vi "HFRR ADV v06.vi"() -> ()   [LabVIEW 2025] (continued)
                  n763 = property class="Instr"(reference=w1044, error in=w1045) -> (reference out=w1049:refnum<visa-resource-name>, error out=w1048:errorcluster, "Serial Settings:Number of Bytes at Serial Port"=w1040:u32)
                  n764 = VISA Read(VISA resource name=w1049, byte count=w1040, error in (no error)=w1048) -> (VISA resource name out=w1046:refnum<visa-resource-name>, read buffer=w1038:string, error out=w1047:errorcluster)  [unwired: 1 out]
                  n765 = Greater?(x=w1040, y=u32 30) -> (0:w1042:bool)
                  n766 = Concatenate Strings(w1039, w1038) -> (w1037:string)
                }
                "UnoRead" <- w989
                n767 = while {
                  shift-right: [w1023] -> w1000
                  shift-left: w989 -> [w1029]
                  tunnel: [w1022] -> w996 mode=indexing
                  tunnel: [w1024] -> _
                  i -> [w1024]
                  stop <- w1026 stop-if-true
                  n768 = Match Pattern(string=w1029, regular expression="*") -> (after substring=w1027:string)  [unwired: 1 in, 3 out]
                  n769 = Match Pattern(string=w1027, regular expression="&") -> (before substring=w1022:string, after substring=w1023:string, offset past match=w1025:i32)  [unwired: 1 in, 1 out]
                  n770 = Less Than 0?(x=w1025) -> (x < 0?=w1026:bool)
                }
                n771 = local write "Residual Uno"(w1000) -> ()
                n772 = Array Size(array=w996) -> (size(s)=w997:i32)
                n773 = Decrement(x=w997) -> (x-1=w999:i32)
                n774 = Delete From Array(array=w996, length=1, index=w999) -> (array with subset deleted=w994:string[])  [unwired: 1 out]
                n775 = Array Size(array=w994) -> (size(s)=w993:i32)
                n776 = Decrement(x=w993) -> (x-1=w992:i32)
                n777 = while {
                  tunnel: [w1021] -> w1005 mode=indexing
                  tunnel: [w1020] -> w1004 mode=indexing
                  tunnel: w994 -> [w1014] mode=indexing
                  tunnel: w992 -> [w1013]
                  tunnel: [w1011] -> _
                  i -> [w1011]
                  stop <- w1012 stop-if-true
                  w1015 = 0 ("length (rest)")
                  w1017 = ";" ("regular expression")
                  n778 = Less Or Equal?(x=w1013, y=w1011) -> (x <= y?=w1012:bool)
                  n779 = Match Pattern(string=w1014, regular expression=w1017) -> (before substring=w1019:string, after substring=w1018:string)  [unwired: 1 in, 2 out]
                  n780 = Decimal String To Number(string=w1019, default (0L)=w1015) -> (number=w1021:i32)  [unwired: 1 in, 1 out]
                  n781 = Match Pattern(string=w1018, regular expression=w1017) -> (before substring=w1016:string)  [unwired: 1 in, 3 out]
                  n782 = Decimal String To Number(string=w1016, default (0L)=w1015) -> (number=w1020:i32)  [unwired: 1 in, 1 out]
                }
                n783 = case shown="0, Default" "ADC Res" {
                  tunnel: [w1032 w1034] -> w988
                  frame 0, Default {
                    n784 = Divide(x=65535 ("length (rest)"), y=2 ("length (rest)")) -> (x/y=w1032:dbl)
                  }
                  frame 1 {
                    n785 = Divide(x=16777216 ("length (rest)"), y=2 ("length (rest)")) -> (x/y=w1034:dbl)
                  }
                }
                n786 = Bundle(w1005, w1004) -> (w995:cluster{i32[], i32[]})  [unwired: 1 in]
                n787 = Divide(x=w995, y=w988) -> (x/y=w1006:cluster{dbl[], dbl[]})
                n788 = Multiply(x=w1006, y=sgl 5.03 ("Numeric")) -> (x*y=w1003:cluster{dbl[], dbl[]})
                n789 = Unbundle(w1003) -> (→"Ch1":dbl[], →"Ch0":dbl[])
              }
            }
            n790 = Not(x=w977) -> (.not. x?=→"Port 1a":bool)
          }
          frame #1 {
            n791 = local read "zOff 2"() -> (w1084:dbl)
            n792 = local read "Ch1"() -> (w1074:dbl[])
            n793 = case shown="True" "Zero 2" {
              tunnel: w1074 -> [_ w1104]
              frame False {
              }
              frame True {
                n794 = call-poly <vilib>:"Mean.vi"("X"=w1104) -> ("mean"=→"zOff 2":dbl)  [unwired: 1 out]
                n795 = local write "Zero 2"(FALSE ("Zero")) -> ()
              }
            }
            n796 = Subtract(x=w1074, y=w1084) -> (x-y=w1080:dbl[])
            n797 = call-poly <vilib>:"Mean.vi"("X"=w1074) -> ("mean"=w1075:dbl)  [unwired: 1 out]
            "Slide 3" <- w1075
            n798 = Multiply(x=w1080, y=1.0 ("PG Oth")) -> (x*y=w1066:dbl[])
            n799 = local read "FF buffer"() -> (w1071:dbl[])
            n800 = Divide(x=w1066, y=1) -> (x/y=w1065:dbl[])
            "Fric Val" <- w1065
            n801 = call <vilib>:"Mean PtByPt.vi"("x"=w1075, "sample length"=10, "initialize"="Reset 2") -> ("mean"=→"Mean Pos Fil 2":dbl)  [unwired: 1 in, 1 out]
            n802 = Array Size(array=w1071) -> (size(s)=w1073:i32)
            n803 = call-poly <vilib>:"Mean.vi"("X"=w1065) -> ("mean"=w1079:dbl)  [unwired: 1 out]
            n804 = Insert Into Array(array=w1071, index=w1073, new element=w1065) -> (w1068:dbl[])
            n805 = Array Size(array=w1068) -> (size(s)=w1067:i32)
            n806 = case shown="True" "DC corr 2" {
              tunnel: w1065 -> [w1107 w1110]
              tunnel: [w1107 w1109] -> w1072
              tunnel: w1079 -> [_ w1108]
              frame False {
              }
              frame True {
                n807 = Subtract(x=w1110, y=w1108) -> (x-y=w1109:dbl[])
              }
            }
            n808 = Tick Count (ms)() -> (millisecond timer value=w1091:u32)
            n809 = Greater?(x=w1067, y=1000) -> (0:w1069:bool)
            n810 = Subtract(x=w1091, y=w1092) -> (x-y=w1090:u32)
            n811 = case shown="True" w1069 {
              tunnel: [w1097 w1100] -> w1056
              tunnel: w1068 -> [w1097 w1103]
              tunnel: w1067 -> [_ w1102]
              frame False {
              }
              frame True {
                n812 = Subtract(x=w1102, y=1000) -> (x-y=w1098:i32)
                n813 = Delete From Array(array=w1103, length=w1098, index=0) -> (array with subset deleted=w1100:dbl[])  [unwired: 1 out]
              }
            }
            n814 = Divide(x=w1090, y=u32 1000 ("x")) -> (x/y=w1088:dbl)
            n815 = Array Size(array=w1072) -> (size(s)=w1087:i32)
            n816 = Divide(x=w1087, y=w1088) -> (x/y=w1083:dbl)
            "Sps 2" <- w1083
            n817 = Reciprocal(x=w1083) -> (1/x=w1081:dbl)
            "dt" <- w1081
            n818 = local read "FRIC. FORCE :"() -> (w1053:dbl)
            n819 = local write "FF buffer"(w1056) -> ()
            n820 = Negate(x=w1056) -> (-x=w1055:dbl[])
            n821 = call "Elapsed Time5"("Time Target (s)"="check time s", "Reset"="Reset 3") -> ("Time has Elapsed"=w1058:bool)  [unwired: 10 in, 7 out]
            n822 = Array Max & Min(array=w1055) -> (max value=w1063:dbl)  [unwired: 3 out]
            n823 = Bundle By Name("Y"=w1072, "dt"=w1081, "t0"=timestamp(0 s since 1904-01-01)) -> (w1051:waveform(dbl))  [unwired: 1 in]
            n824 = Multiply(x=w1053, y=21.1986) -> (x*y=w1052:dbl)
            n825 = Greater Or Equal?(x=w1063, y="Threshold value") -> (x >= y?=w1059:bool)
            n826 = Multiply(x=w1052, y=w1051) -> (x*y=→"FF_Wfm":waveform(dbl))
            n827 = And(x=w1059, y=w1058) -> (x .and. y?=w1057:bool)
            n828 = case shown="True" w1057 {
              frame False {
                n829 = local write "Reset 3"(FALSE ("Reset 3")) -> ()
              }
              frame True {
                n830 = local write "Reset 3"(TRUE ("Reset 3")) -> ()
                n831 = local write "save dpt"(TRUE ("save dpt")) -> ()
              }
            }
          }
          frame #2 {
            n832 = local read "FF buffer"() -> (w1117:dbl[])
            n833 = Array Max & Min(array=w1117) -> (max value=w1112:dbl, min value=w1113:dbl)  [unwired: 2 out]
            n834 = Subtract(x=w1112, y=w1113) -> (x-y=w1114:dbl)
            n835 = Multiply(x=1.0 ("y 2"), y="Threshold") -> ()  [unwired: 1 out]
            n836 = Greater?(x=w1114, y="Threshold") -> (0:w1111:bool)
            n837 = case shown="True" w1111 {
              tunnel: w1117 -> [_ w1124]
              tunnel: [_ w1122] -> _
              frame False {
              }
              frame True {
                w1123 = 1.0 ("y")
                n838 = Delete From Array(array=w1124, length=100, index=0) -> (deleted portion=w1129:dbl[])  [unwired: 1 out]
                n839 = call-poly <vilib>:"Mean.vi"("X"=w1129) -> ("mean"=w1128:dbl)  [unwired: 1 out]
                n840 = Subtract(x=w1124, y=w1128) -> (x-y=w1127:dbl[])
                n841 = Multiply(x=w1123, y=w1123) -> (x*y=w1125:dbl)
                n842 = Multiply(x=w1127, y=w1125) -> (x*y=w1126:dbl[])
                "FF cal val" <- w1126
                n843 = Array Size(array=w1126) -> (size(s)=w1120:i32)
                n844 = Array Max & Min(array=w1126) -> (max value=w1119:dbl, min value=w1118:dbl)  [unwired: 2 out]
                n845 = property on="FF Calibration g" class="WFGraph (strict)"("X Scale.Range:Minimum"=0.0 ("y"), "X Scale.Range:Maximum"=w1120, "Y Scale.Range:Minimum"=w1119, "Y Scale.Range:Maximum"=w1118) -> ()  [unwired: 2 in, 2 out]
                n846 = local read "FRIC. FORCE :"() -> (w1122:dbl)
              }
            }
          }
          frame #3 {
            # "5"
            n847 = local read "DISPLACEMENT :"() -> (w1217:dbl)
            n848 = Multiply(x=w1217, y=1.0) -> (x*y=w1134:dbl)
            n849 = local read "zOff 3"() -> (w1220:dbl)
            n850 = local read "Ch0"() -> (w1147:dbl[])
            n851 = case shown="True" "Zero 3" {
              tunnel: w1147 -> [_ w1235]
              frame False {
              }
              frame True {
                n852 = call-poly <vilib>:"Mean.vi"("X"=w1235) -> ("mean"=→"zOff 3":dbl)  [unwired: 1 out]
                n853 = local write "Zero 3"(FALSE ("Zero")) -> ()
              }
            }
            n854 = Add(x=w1147, y="Offset") -> (x+y=w1146:dbl[])
            n855 = Multiply(x=w1134, y="DISPLACEMENT : 2") -> (x*y=w1201:dbl)
            n856 = Subtract(x=w1147, y=w1220) -> (x-y=w1204:dbl[])
            n857 = Multiply(x=w1204, y=w1201) -> (x*y=w1203:dbl[])
            n858 = Multiply(x=w1204, y=w1134) -> (x*y=w1216:dbl[])
            "ABS DP" <- w1216
            n859 = local read "Standard Slip Gauge (mm)"() -> (w1202:dbl)
            n860 = call-poly <vilib>:"Mean.vi"("X"=w1203) -> ("mean"=w1133:dbl)  [unwired: 1 out]
            "Disp (mm)" <- w1133
            "software msrnt" <- w1133
            n861 = Multiply(x=w1146, y="Gain") -> (x*y=w1141:dbl[])
            "Voltage LVDT Acq" <- w1141
            "gLVDTraw" <- w1141
            n862 = call-poly <vilib>:"Mean.vi"("X"=w1216) -> ("mean"=w1206:dbl)  [unwired: 1 out]
            n863 = case shown="True" "DC correction" {
              tunnel: w1216 -> [w1238 w1241]
              tunnel: [w1238 w1240] -> w1153
              tunnel: w1206 -> [_ w1239]
              frame False {
              }
              frame True {
                n864 = Subtract(x=w1241, y=w1239) -> (x-y=w1240:dbl[])
              }
            }
            n865 = Divide(x=w1133, y=w1202) -> (x/y=w1200:dbl)
            n866 = call-poly <vilib>:"Mean.vi"("X"=w1141) -> ("mean"=w1140:dbl)  [unwired: 1 out]
            n867 = Array Max & Min(array=w1141) -> (max value=w1145:dbl, min value=w1144:dbl)  [unwired: 2 out]
            n868 = Multiply(x=w1200, y=w1201) -> (x*y=→"DISPLACEMENT : 3":dbl)
            n869 = Subtract(x=w1145, y=w1144) -> (x-y=→"Pk-Pk":dbl)
            n870 = local read "dt"() -> (w1219:dbl)
            n871 = Threshold 1D Array(2:0.0 ("threshold y"), 3:w1153) -> (0:w1170:dbl)  [unwired: 1 in]
            n872 = Bundle By Name("Y"=w1153, "dt"=w1219, "t0"=timestamp(0 s since 1904-01-01)) -> (w1208:waveform(dbl))  [unwired: 1 in]
            n873 = local read "FF_Wfm"() -> (w1207:waveform(dbl))
            n874 = Equal To 0?(x=w1170) -> (x = 0?=w1171:bool)
            n875 = case shown="True" w1171 {
              tunnel: w1153 -> [_ w1229]
              tunnel: [w1225 w1226] -> w1166
              tunnel: w1170 -> [w1225 _]
              frame False {
              }
              frame True {
                n876 = Threshold 1D Array(1:20 ("start index (0)"), 2:0.0 ("threshold y"), 3:w1229) -> (0:w1226:dbl)
              }
            }
            n877 = call-poly <vilib>:"Extract Single Tone Information.vi"("time signal in"=w1208) -> ("detected amplitude"=w1142:dbl, "detected frequency"=→"Freq":dbl)  [unwired: 5 in, 4 out]
            n878 = Build Array(w1208, w1207) -> (w1189:waveform(dbl)[])
            "Waveform Graph 2" <- w1189
            n879 = Subtract(x=w1140, y="LvdtOff") -> (x-y=w1139:dbl)
            n880 = Subtract(x=w1139, y=w1142) -> (x-y=w1151:dbl)
            n881 = Add(x=w1142, y=w1139) -> (x+y=w1150:dbl)
            n882 = Index Array(array=w1189) -> (element #1=w1190:waveform(dbl), element #2=w1192:waveform(dbl))  [unwired: 2 in]
            n883 = Multiply(x=w1142, y=2.0) -> (x*y=w1209:dbl)
            "Stroke" <- w1209
            "Mean(RAW) Stroke" <- w1209
            n884 = Bundle(w1139, w1151, w1150) -> (→"Slide 8":cluster{dbl, dbl, dbl})  [unwired: 1 in]
            n885 = Unbundle By Name(w1190) -> ("Y"=w1163:dbl[])
            n886 = Split 1D Array(array=w1153, index=w1166) -> (second subarray=w1167:dbl[])  [unwired: 1 out]
            n887 = In Range and Coerce(upper limit=1.5, x=w1209, lower limit=0.5) -> (In Range?=w1213:bool)  [unwired: 1 out]
            n888 = Split 1D Array(array=w1163, index="Window") -> (second subarray=w1181:dbl[])  [unwired: 1 out]
            n889 = Unbundle By Name(w1192) -> ("Y"=w1164:dbl[])
            n890 = Threshold 1D Array(1:180 ("start index (0)"), 2:0.0 ("threshold y"), 3:w1167) -> (0:w1165:dbl)
            n891 = local read "Test \nStatus"() -> (w1210:bool)
            n892 = Split 1D Array(array=w1164, index=w1166) -> (second subarray=w1161:dbl[])  [unwired: 1 out]
            n893 = Not(x=w1213) -> (.not. x?=w1212:bool)
            n894 = call-poly <vilib>:"RMS.vi"("X"=w1181) -> ("rms value"=w1137:dbl)  [unwired: 1 out]
            "Current (A)" <- w1137
            n895 = Array Max & Min(array=w1181) -> (max value=w1195:dbl, min value=w1196:dbl)  [unwired: 2 out]
            n896 = Array Max & Min(array=w1164) -> (max value=w1193:dbl, min value=w1194:dbl)  [unwired: 2 out]
            n897 = Subtract(x=w1195, y=w1196) -> (x-y=w1197:dbl)
            n898 = Subtract(x=w1193, y=w1194) -> (x-y=w1198:dbl)
            n899 = And(x=w1212, y=w1210) -> (x .and. y?=w1211:bool)
            n900 = Split 1D Array(array=w1167, index=w1165) -> (first subarray=w1160:dbl[])  [unwired: 1 out]
            n901 = Split 1D Array(array=w1161, index=w1165) -> (first subarray=w1158:dbl[])  [unwired: 1 out]
            n902 = case shown="True" w1211 {
              tunnel: [i32[] [] w1231] -> _
              frame False {
              }
              frame True {
                n903 = local read "UnoRead"() -> (w1233:string)
                n904 = local read "Array"() -> (w1234:string[])
                n905 = Build Array (concatenate)(w1234, w1233) -> (w1232:string[])
                "Array" <- w1232
                n906 = String Length(string=w1232) -> (length=w1231:i32[])
              }
            }
            n907 = local read "G_val"() -> (w1183:dbl)
            n908 = Divide(x=w1198, y=w1197) -> (x/y=w1186:dbl)
            n909 = call-poly <vilib>:"RMS.vi"("X"=w1158) -> ("rms value"=w1182:dbl)  [unwired: 1 out]
            n910 = call-poly <vilib>:"Hanning Window.vi"("X"=w1160) -> ("Windowed X"=w1159:dbl[])  [unwired: 1 out]
            n911 = call-poly <vilib>:"Hanning Window.vi"("X"=w1158) -> ("Windowed X"=w1157:dbl[])  [unwired: 1 out]
            n912 = local read "Constant (G)"() -> (w1175:dbl)
            n913 = Divide(x=w1182, y=w1137) -> (x/y=w1176:dbl)
            n914 = Build Array(w1159, w1157) -> (→"Waveform Graph 4":dbl[][])
            n915 = Multiply(x=w1186, y=0.2) -> (x*y=w1188:dbl)
            n916 = Multiply(x=0.8 ("y"), y=w1183) -> (x*y=w1187:dbl)
            n917 = Add(x=w1188, y=w1187) -> (x+y=w1155:dbl)
            n918 = Multiply(x=w1176, y=0.2) -> (x*y=w1177:dbl)
            n919 = Multiply(x=0.8 ("y"), y=w1175) -> (x*y=w1178:dbl)
            n920 = Add(x=w1177, y=w1178) -> (x+y=w1174:dbl)
            "Constant (G)" <- w1174
            n921 = Not A Number/Path/Refnum?(number/path/refnum=w1155) -> (NaN/Path/Refnum?=w1154:bool)
            n922 = Select(t=0.0, s=w1154, f=w1155) -> (s? t:f=w1135:dbl)
            "G_val" <- w1135
            n923 = Multiply(x=w1137, y=w1135) -> (x*y=→"Friction Force (N)":dbl)
            n924 = Bundle(w1174, "t"=w1135) -> (→"pk-pk":cluster{dbl, "t":dbl})  [unwired: 1 in]
          }
          frame #4 {
            # "C:\\WinDucom\\data\\"
            # "?C:\\LAB-IQ-NXT\\data"
            n925 = case shown="True" "save dpt" {
              frame False {
              }
              frame True {
                n926 = local write "save dpt"(FALSE ("Hold 3")) -> ()
                n927 = local read "file count"() -> (w1245:i32)
                n928 = Number To Decimal String(number=w1245) -> (decimal integer string=w1251:string)  [unwired: 1 in]
                n929 = Add(x=1, y=w1245) -> (x+y=w1246:i32)
                n930 = local write "file count"(w1246) -> ()
                n931 = local read "FILE 2"() -> (w1250:string)
                n932 = Concatenate Strings(w1250, w1251) -> (w1243:string)
                n933 = Concatenate Strings("C:\\LAB-IQ\\data" ("Substring"), w1243) -> (w1258:string)
                n934 = local read "FF buffer"() -> (w1253:dbl[])
                n935 = local read "ABS DP"() -> (w1252:dbl[])
                n936 = Concatenate Strings(w1258, ".dpf" ("Substring")) -> (w1256:string)
                n937 = Build Array(w1253, w1252) -> (w1248:dbl[][])
                n938 = Concatenate Strings("FF ( V ); DP( mincron ) " ("character string"), "\r") -> (w1262:string)
                n939 = String To Path(string=w1256) -> (path=w1254:path)
                n940 = Transpose 2D Array(2D array=w1248) -> (transposed array=w1247:dbl[][])
                n941 = call <vilib>:"Write Characters To File.vi"("append to file? (new file:F)"=FALSE, "character string"=w1262, "file path (dialog if empty)"=w1254) -> ("new file path (Not A Path if cancelled)"=w1259:path)  [unwired: 2 in]
                n942 = Array To Spreadsheet String(delimiter (Tab)=";", array=w1247, 3:"" ("format string")) -> (spreadsheet string=w1249:string)
                "String 9" <- w1249
                n943 = call <vilib>:"Write Characters To File.vi"("append to file? (new file:F)"=TRUE, "character string"=w1249, "file path (dialog if empty)"=w1259) -> ()  [unwired: 2 in, 1 out]
              }
            }
          }
          frame #5 {
            n944 = case shown="True" "Hold 4" {
              frame False {
              }
              frame True {
                n945 = File Dialog(6:"*.dpf" ("pattern"), 11:path "C:/LAB-IQ" ("start path")) -> (0:w1269:errorcluster, 3:w1284:path)  [unwired: 5 in, 2 out]
                n946 = Unbundle(w1269) -> ()  [unwired: 3 out]
                n947 = call <vilib>:"Read Characters From File.vi"("file path (dialog if empty)"=w1284) -> ("character string"=w1274:string)  [unwired: 5 in, 3 out]
                n948 = Spreadsheet String To Array(delimiter (Tab)=";", format string="%S", spreadsheet string=w1274, array type (2D Dbl)=string[][] []) -> (array=w1278:string[][])
                n949 = for {
                  tunnel: w1278 -> [w1288] mode=indexing
                  tunnel: [w1287] -> w1279 mode=indexing
                  n950 = for {
                    tunnel: w1288 -> [w1290] mode=indexing
                    tunnel: [w1289] -> w1287 mode=indexing
                    n951 = call <vilib>:"Trim Whitespace.vi"("string"=w1290) -> ("trimmed string"=w1289:string)  [unwired: 1 in]
                  }
                }
                n952 = Fract/Exp String To Number(string=w1279) -> (number=w1281:dbl[][])  [unwired: 3 in, 1 out]
                n953 = Array Subset(array=w1281, index (row)=1 ("index (col)")) -> (w1283:dbl[][])  [unwired: 3 in]
                n954 = Index Array(array=w1283, index (col) #1=0 ("disabled index (col)"), index (col) #2=1 ("disabled index (col)")) -> (element #1=w1272:dbl[], element #2=w1271:dbl[])  [unwired: 2 in]
                n955 = Build Array(w1272, w1271) -> (→"Waveform Graph":dbl[][])
              }
            }
          }
        }
      }
      frame Error {
        w1306 = u16 0 items=["None", "XON/XOFF", "RTS/CTS", "XON/XOFF & RTS/CTS", "DTR/DSR", "XON/XOFF & DTR/DSR"] ("flow control (0:none)  2")
        w1304 = u16 10 items=["1.0"=10, "1.5"=15, "2.0"=20] ("stop bits 2")
        w1302 = u16 0 items=["None", "Odd", "Even", "Mark", "Space"] ("parity 2")
        w1303 = u32 10000  # timeout (10sec)
        n956 = VISA Close(VISA resource name=w1298, error in (no error)=w1295) -> (error out=w1299:errorcluster)
        n957 = local write "Sps 3"(0.0 ("Sps 4")) -> ()
        n958 = call <vilib>:"Clear Errors.vi"("error in (no error)"=w1299) -> ("error out"=w1296:errorcluster)  [unwired: 5 in, 1 out]
        n959 = local read "Com Port 1"() -> (w1291:refnum<visa-resource-name>)
        n960 = call-poly "VISA Configure Serial Port"("VISA resource name"=w1291, "timeout (10sec)"=w1303, "baud rate (9600)"=u32 250000 ("baud rate  2"), "data bits (8)"=u16 8 ("data bits  2"), "parity (0:none)"=w1302, "error in (no error)"=w1296, "stop bits (10: 1 bit)"=w1304, "flow control (0:none)"=w1306) -> ("VISA resource name out"=w1307:refnum<visa-resource-name>, "error out"=w1308:errorcluster)  [unwired: 6 in]
        n961 = flat-sequence {
          tunnel: w1307 -> [w1310]
          tunnel: w1308 -> [w1309]
          tunnel: [w1310] -> w1300
          tunnel: [w1309] -> w1292
          frame #0 {
            n962 = Wait (ms)(milliseconds to wait=u32 50) -> ()  [unwired: 1 out]
          }
        }
        "Residual Uno" <- ""
        "Port 1 Error" <- w1292
      }
    }
    n963 = local read "Quit"() -> (w945:bool)
    "Error Uno" <- w953
  }
  n964 = while {
    shift-right: [w1327] -> w25
    shift-left: _ -> [w1318]
    shift-right: [w1326] -> w24
    shift-left: errorcluster {"status"=FALSE, "code"=0, "source"="Init"} ("error out") -> [w1320]
    tunnel: [w1312] -> w30
    tunnel: [w1325] -> _
    i -> [w1325]
    stop <- w1312 stop-if-true
    n965 = local read "Com Port 2"() -> (w1319:refnum<visa-resource-name>)
    n966 = local read "Port 2a"() -> (w1321:bool)
    n967 = local read "Port 4"() -> (w1322:bool)
    n968 = Not Equal?(x=w1319, y=w1318) -> (x != y?=w1317:bool)
    n969 = Or(x=w1322, y=w1321) -> (x .or. y?=w1324:bool)
    n970 = Unbundle(w1320) -> ("status"=→"Port 4":bool)  [unwired: 2 out]
    n971 = flat-sequence {
      tunnel: w1320 -> [w1331]
      tunnel: [w1331] -> w1316
      frame #0 {
        n972 = Wait (ms)(milliseconds to wait=u32 50) -> ()  [unwired: 1 out]
      }
    }
    n973 = local read "Re-Initialise"() -> (w1313:bool)
    n974 = case shown="True" w1324 {
      frame False {
        w1332 = FALSE ("Visible")
        n975 = property on="Port 2a" class="Bool (strict)"("Visible"=w1332) -> ()  [unwired: 2 in, 2 out]
        n976 = property on="Port 4" class="Bool (strict)"("Visible"=w1332) -> ()  [unwired: 2 in, 2 out]
      }
      frame True {
        w1333 = TRUE ("Visible")
        n977 = property on="Port 2a" class="Bool (strict)"("Visible"=w1333) -> ()  [unwired: 2 in, 2 out]
        n978 = property on="Port 4" class="Bool (strict)"("Visible"=w1333) -> ()  [unwired: 2 in, 2 out]
      }
    }
    n979 = Or(x=w1317, y=w1313) -> (x .or. y?=w1314:bool)
    n980 = case shown="True" w1314 {
      tunnel: [w1328 errorcluster {"status"=TRUE, "code"=0, "source"="Init"} ("error out")] -> w1315
      tunnel: w1316 -> [w1328 _]
      frame False {
      }
      frame True {
      }
    }
    n981 = case shown="Error" w1315 {
      selector: w1315 -> [w1334 w1488]
      tunnel: [w1336 w1493] -> w1327
      tunnel: [w1335 w1486] -> w1326
      tunnel: w1318 -> [w1338 w1491]
      tunnel: [w1337 _] -> _
      frame No Error {
        n982 = stacked-sequence {
          tunnel: w1338 -> [w1362 _]
          tunnel: w1334 -> [w1361 _]
          tunnel: [w1348 _] -> w1337
          tunnel: [w1347 _] -> w1336
          tunnel: [w1346 _] -> w1335
          frame #0 {
            n983 = property class="Instr"(reference=w1362, error in=w1361) -> (reference out=w1345:refnum<visa-resource-name>, error out=w1360:errorcluster, "Serial Settings:Number of Bytes at Serial Port"=w1341:u32)
            "Port 2" <- w1341
            n984 = Greater?(x=w1341, y=u32 23) -> (0:w1343:bool)
            n985 = Not(x=w1343) -> ()  [unwired: 1 out]
            n986 = case shown="True" w1343 {
              tunnel: w1345 -> [w1377 w1402]
              tunnel: w1360 -> [w1376 w1403]
              tunnel: [w1376 w1405] -> w1356
              tunnel: [w1377 w1404] -> w1357
              frame False {
              }
              frame True {
                # "Out as Volts"
                n987 = local read "Residual Due"() -> (w1401:string)
                n988 = while {
                  tunnel: [w1445] -> w1405
                  tunnel: [w1444] -> w1404
                  tunnel: w1403 -> [w1443]
                  tunnel: w1402 -> [w1442]
                  tunnel: [w1439] -> _
                  shift-right: [w1437] -> w1400
                  shift-left: w1401 -> [w1436]
                  i -> [w1439]
                  stop <- w1440 stop-if-true
                  n989 = property class="Instr"(reference=w1442, error in=w1443) -> (reference out=w1447:refnum<visa-resource-name>, error out=w1446:errorcluster, "Serial Settings:Number of Bytes at Serial Port"=w1438:u32)
                  n990 = VISA Read(VISA resource name=w1447, byte count=w1438, error in (no error)=w1446) -> (VISA resource name out=w1444:refnum<visa-resource-name>, read buffer=w1435:string, error out=w1445:errorcluster)  [unwired: 1 out]
                  n991 = Greater?(x=w1438, y=u32 8) -> (0:w1440:bool)
                  n992 = Concatenate Strings(w1436, w1435) -> (w1437:string)
                }
                n993 = while {
                  shift-right: [w1428] -> w1384
                  shift-left: w1400 -> [w1433]
                  tunnel: [w1427] -> w1396 mode=indexing
                  tunnel: [w1426] -> _
                  i -> [w1426]
                  stop <- w1430 stop-if-true
                  n994 = Match Pattern(string=w1433, regular expression="*") -> (after substring=w1431:string)  [unwired: 1 in, 3 out]
                  n995 = Match Pattern(string=w1431, regular expression="&") -> (before substring=w1427:string, after substring=w1428:string, offset past match=w1429:i32)  [unwired: 1 in, 1 out]
                  n996 = Less Than 0?(x=w1429) -> (x < 0?=w1430:bool)
                }
                n997 = Array Size(array=w1396) -> (size(s)=w1399:i32)
                n998 = local write "Residual Due"(w1384) -> ()
                n999 = Decrement(x=w1399) -> (x-1=w1397:i32)
                n1000 = Delete From Array(array=w1396, length=1, index=w1397) -> (array with subset deleted=w1395:string[])  [unwired: 1 out]
                n1001 = Array Size(array=w1395) -> (size(s)=w1383:i32)
                n1002 = Decrement(x=w1383) -> (x-1=w1382:i32)
                n1003 = while {
                  tunnel: w1395 -> [w1414] mode=indexing
                  tunnel: w1382 -> [w1413]
                  tunnel: [w1411] -> w1390 mode=indexing
                  tunnel: [w1410] -> w1389 mode=indexing
                  tunnel: [w1409] -> w1388 mode=indexing
                  tunnel: [w1408] -> w1387 mode=indexing
                  tunnel: [w1407] -> w1385 mode=indexing
                  tunnel: [w1406] -> _
                  i -> [w1406]
                  stop <- w1412 stop-if-true
                  w1423 = u32 0 ("length (rest)")
                  w1422 = ";" ("regular expression")
                  n1004 = Less Or Equal?(x=w1413, y=w1406) -> (x <= y?=w1412:bool)
                  n1005 = Match Pattern(string=w1414, regular expression=w1422) -> (before substring=w1415:string, after substring=w1416:string)  [unwired: 1 in, 2 out]
                  n1006 = Match Pattern(string=w1416, regular expression=w1422) -> (before substring=w1419:string, after substring=w1417:string)  [unwired: 1 in, 2 out]
                  n1007 = Decimal String To Number(string=w1415, default (0L)=w1423) -> (number=w1411:u32)  [unwired: 1 in, 1 out]
                  n1008 = Decimal String To Number(string=w1419, default (0L)=w1423) -> (number=w1410:u32)  [unwired: 1 in, 1 out]
                  n1009 = Match Pattern(string=w1417, regular expression=w1422) -> (before substring=w1420:string, after substring=w1418:string)  [unwired: 1 in, 2 out]
                  n1010 = Decimal String To Number(string=w1420, default (0L)=w1423) -> (number=w1409:u32)  [unwired: 1 in, 1 out]
                  n1011 = Match Pattern(string=w1418, regular expression=w1422) -> (before substring=w1421:string, after substring=w1425:string)  [unwired: 1 in, 2 out]
                  n1012 = Decimal String To Number(string=w1421, default (0L)=w1423) -> (number=w1408:u32)  [unwired: 1 in, 1 out]
                  n1013 = Decimal String To Number(string=w1425, default (0L)=u8 0 ("length (rest)")) -> (number=w1407:u8)  [unwired: 1 in, 1 out]
                }
                "Din" <- w1385
                n1014 = Bundle(w1390, w1389, w1388, w1387) -> (w1392:cluster{u32[], u32[], u32[], u32[]})  [unwired: 1 in]
                n1015 = Divide(x=w1392, y=4095 ("length (rest)")) -> (x/y=w1394:cluster{dbl[], dbl[], dbl[], dbl[]})
                n1016 = Multiply(x=w1394, y=sgl 3.32 ("Numeric")) -> (x*y=w1386:cluster{dbl[], dbl[], dbl[], dbl[]})
                n1017 = Unbundle(w1386) -> (→"ECR":dbl[], →"Rtemp":dbl[], →"Air temp":dbl[], →"Ch3 2":dbl[])
              }
            }
            n1018 = call "Elapsed Time10"("Time Target (s)"=2.0, "Reset"=w1343, "Auto Reset"=FALSE) -> ("Time has Elapsed"=→"Port 2a":bool)  [unwired: 9 in, 7 out]
            n1019 = local read "Due Com"() -> (w1349:string[])
            n1020 = Array Size(array=w1349) -> (size(s)=w1348:i32)
            n1021 = Delete From Array(array=w1349, length=1, index=0) -> (deleted portion=w1352:string[], array with subset deleted=w1353:string[])
            n1022 = local write "Due Com"(w1353) -> ()
            n1023 = Index Array(array=w1352, index=0) -> (element=w1350:string)
            n1024 = Not Equal?(x=w1350, y="") -> (x != y?=w1358:bool)
            n1025 = case shown="True" w1358 {
              tunnel: w1357 -> [w1364 w1369]
              tunnel: [w1364 w1373] -> w1347
              tunnel: w1356 -> [w1363 w1368]
              tunnel: [w1363 w1371] -> w1346
              tunnel: w1350 -> [_ w1367]
              tunnel: [_ w1370] -> _
              frame False {
                # "DATA  WRITE LOOP"
              }
              frame True {
                n1026 = Concatenate Strings(w1367, "\r\n") -> (w1366:string)
                n1027 = VISA Write(VISA resource name=w1369, write buffer=w1366, error in (no error)=w1368) -> (VISA resource name out=w1373:refnum<visa-resource-name>, return count=w1370:u32, error out=w1372:errorcluster)
                n1028 = flat-sequence {
                  tunnel: w1372 -> [w1374]
                  tunnel: [w1374] -> w1371
                  frame #0 {
                    n1029 = Wait (ms)(milliseconds to wait=u32 5) -> ()  [unwired: 1 out]
                  }
                }
              }
            }
          }
          frame #1 {
            w1456 = 10 ("y")
            w1461 = 10 ("y")
            n1030 = local read "Rtemp"() -> (w1449:dbl[])
            n1031 = local read "ecr buf"() -> (w1450:dbl[])
            n1032 = for {
              tunnel: w1449 -> [w1473] mode=indexing
              shift-right: [w1474] -> w1457
              shift-left: dbl[] [] ("temp buf 2") -> [w1475]
              n1033 = Build Array (concatenate)(w1475, w1473) -> (w1476:dbl[])
              n1034 = Equal To 0?(x=w1473) -> (x = 0?=w1477:bool)
              n1035 = Select(t=w1475, s=w1477, f=w1476) -> (s? t:f=w1474:dbl[])
            }
            n1036 = local read "ECR"() -> (w1448:dbl[])
            n1037 = Insert Into Array(array=w1448, index=0, new element=w1450) -> (w1454:dbl[])
            n1038 = local read "temp buf"() -> (w1458:dbl[])
            n1039 = Array Size(array=w1454) -> (size(s)=w1455:i32)
            n1040 = Greater?(x=w1455, y=w1456) -> (0:w1453:bool)
            n1041 = case shown="True" w1453 {
              tunnel: w1454 -> [w1466 w1472]
              tunnel: w1455 -> [_ w1470]
              tunnel: w1456 -> [_ w1469]
              tunnel: [w1466 w1467] -> w1451
              frame False {
              }
              frame True {
                n1042 = Subtract(x=w1470, y=w1469) -> (x-y=w1468:i32)
                n1043 = Delete From Array(array=w1472, length=w1468, index=0) -> (array with subset deleted=w1467:dbl[])  [unwired: 1 out]
              }
            }
            "ecr buf" <- w1451
            n1044 = Insert Into Array(array=w1457, index=0, new element=w1458) -> (w1463:dbl[])
            n1045 = Array Size(array=w1463) -> (size(s)=w1462:i32)
            n1046 = Greater?(x=w1462, y=w1461) -> (0:w1464:bool)
            n1047 = case shown="True" w1464 {
              tunnel: w1463 -> [w1478 w1484]
              tunnel: w1462 -> [_ w1482]
              tunnel: w1461 -> [_ w1481]
              tunnel: [w1478 w1479] -> w1460
              frame False {
              }
              frame True {
                n1048 = Subtract(x=w1482, y=w1481) -> (x-y=w1480:i32)
                n1049 = Delete From Array(array=w1484, length=w1480, index=0) -> (array with subset deleted=w1479:dbl[])  [unwired: 1 out]
              }
            }
            "temp buf" <- w1460
          }
        }
      }
      frame Error {
        w1499 = u16 0 items=["None", "XON/XOFF", "RTS/CTS", "XON/XOFF & RTS/CTS", "DTR/DSR", "XON/XOFF & DTR/DSR"] ("flow control (0:none)  2")
        w1497 = u16 10 items=["1.0"=10, "1.5"=15, "2.0"=20] ("stop bits 2")
        w1495 = u16 0 items=["None", "Odd", "Even", "Mark", "Space"] ("parity 2")
        w1496 = u32 10000  # timeout (10sec)
        n1050 = VISA Clear(VISA resource name=w1491, error in (no error)=w1488) -> (VISA resource name out=w1490:refnum<visa-resource-name>, error out=w1489:errorcluster)
        n1051 = VISA Close(VISA resource name=w1490, error in (no error)=w1489) -> (error out=w1492:errorcluster)
        n1052 = call <vilib>:"Clear Errors.vi"("error in (no error)"=w1492) -> ()  [unwired: 5 in, 2 out]
        n1053 = local read "Com Port 2"() -> (w1485:refnum<visa-resource-name>)
        "visa due" <- w1485
        n1054 = call-poly "VISA Configure Serial Port"("VISA resource name"=w1485, "timeout (10sec)"=w1496, "baud rate (9600)"=u32 250000 ("baud rate  2"), "data bits (8)"=u16 8 ("data bits  2"), "parity (0:none)"=w1495, "stop bits (10: 1 bit)"=w1497, "flow control (0:none)"=w1499) -> ("VISA resource name out"=w1500:refnum<visa-resource-name>, "error out"=w1501:errorcluster)  [unwired: 7 in]
        n1055 = flat-sequence {
          tunnel: w1500 -> [w1503]
          tunnel: w1501 -> [w1502]
          tunnel: [w1503] -> w1493
          tunnel: [w1502] -> w1486
          frame #0 {
            n1056 = Wait (ms)(milliseconds to wait=u32 50) -> ()  [unwired: 1 out]
          }
        }
        "Residual Due" <- ""
        "Port 2 Error" <- w1486
      }
    }
    n1057 = local read "Quit"() -> (w1312:bool)
    "Error Due" <- w1320
  }
  n1058 = property on="RUN" class="Bool (strict)"("Visible"=TRUE) -> ()  [unwired: 2 in, 2 out]
  n1059 = while {
    tunnel: [w1521] -> _
    tunnel: [w1505] -> w46
    i -> [w1521]
    stop <- w1505 stop-if-true
    n1060 = local read "conststatus"() -> (w1509:dbl)
    n1061 = local read "Main Tab"() -> (w1507:T2)
    n1062 = local read "EDIT"() -> (w1527:bool)
    n1063 = local read "Rate"() -> (w1526:dbl)
    n1064 = case shown="True" w1527 {
      tunnel: [FALSE TRUE] -> w1513
      frame False {
      }
      frame True {
      }
    }
    n1065 = property on="Time slide" class="Slide (strict)"("Scale.Range:Maximum"=2500.0) -> ()  [unwired: 2 in, 2 out]
    n1066 = Equal?(x=w1507, y=T18."About" ("Main Tab")) -> (x = y?=w1519:bool)
    n1067 = Equal?(x=w1509, y=0.0) -> (x = y?=w1510:bool)
    n1068 = Divide(x=1.0, y=w1526) -> (x/y=w1522:dbl)
    "Time 2" <- w1522
    n1069 = case shown="True" w1510 {
      frame False {
      }
      frame True {
        # "C:\\WinDucom\\calibrate WO 2391.dcf"
        n1070 = local write "Lan flag"(22) -> ()
        n1071 = local write "conststatus"(10.0 ("rpm value : 2")) -> ()
        n1072 = String To Path(string="C:\\LAB-IQ\\calibrate WO 2464.dcf") -> (path=w1533:path)
        n1073 = Open/Create/Replace File "Open File"(file path (use dialog)=w1533) -> (refnum out=w1531:refnum<file>)  [unwired: 5 in, 2 out]
        n1074 = for {
          N: 23 -> [_]
          tunnel: w1531 -> [w1542]
          i -> [w1536]
          (unwired) TRUE ("line mode (F)")
          n1075 = Read from Text File "Read File"(file (use dialog)=w1542) -> (text=w1541:string)  [unwired: 3 in, 3 out]
          n1076 = Match Pattern(string=w1541, regular expression="]") -> (after substring=w1539:string)  [unwired: 1 in, 3 out]
          n1077 = String Subset(string=w1541, offset (0)=5, length (rest)=10 ("length (rest)")) -> (substring=w1534:string)
          n1078 = Fract/Exp String To Number(string=w1534) -> (number=w1535:dbl)  [unwired: 3 in, 1 out]
          n1079 = Match Pattern(string=w1539, regular expression="-") -> (before substring=w1537:string)  [unwired: 1 in, 3 out]
          n1080 = case shown="6" w1536 {
            tunnel: w1535 -> [w1545 w1546 w1547 w1548 _ _ _ w1553 w1554 w1555 w1558 w1559 w1560 w1561 w1562 w1563 w1564 w1567 w1568 _ _ w1571 _ _]
            tunnel: w1537 -> [_ _ _ _ w1549 w1550 w1551 _ _ _ _ _ _ _ _ _ _ _ _ w1569 w1570 _ w1572 _]
            frame 0 {
              n1081 = local write "FRIC. FORCE :"(w1545) -> ()
            }
            frame 1 {
              n1082 = local write "TEMPERATURE :"(w1546) -> ()
            }
            frame 2 {
              n1083 = local write "HUMIDITY:"(w1547) -> ()
            }
            frame 3 {
              n1084 = local write "AIR TEMPERATURE :"(w1548) -> ()
            }
            frame 4 {
              n1085 = local write "Com Port 1"(w1549) -> ()
            }
            frame 5 {
              n1086 = local write "Com Port 2"(w1550) -> ()
              n1087 = local write "visa due"(w1550) -> ()
            }
            frame 6 {
              n1088 = String To Path(string=w1551) -> (path=w1552:path)
              n1089 = local write "File Path"(w1552) -> ()
              "String" <- w1551
            }
            frame 7 {
              n1090 = local write "DISPLACEMENT :"(w1553) -> ()
            }
            frame 8 {
              n1091 = local write "STROKE GAIN :"(w1554) -> ()
            }
            frame 9 {
              n1092 = local read "Stroke PID Gains"() -> (w1557:T8)
              n1093 = Bundle By Name(cluster=w1557, "Proportional Gain (Kc)"=w1555) -> (w1556:T8)
              n1094 = local write "Stroke PID Gains"(w1556) -> ()
            }
            frame 10 {
              n1095 = local write "Language Selection"(w1558) -> ()
            }
            frame 11 {
              n1096 = local write "CH-POWER +"(w1559) -> ()
            }
            frame 12 {
              n1097 = local write "CH-POWER -"(w1560) -> ()
            }
            frame 13 {
              n1098 = local write "CH-HEATER"(w1561) -> ()
            }
            frame 14 {
              n1099 = local write "CH-HUMIDITY WET"(w1562) -> ()
            }
            frame 15 {
              n1100 = local write "CH-HUMIDITY DRY"(w1563) -> ()
            }
            frame 16 {
              n1101 = local read "Stroke PID Gains"() -> (w1566:T8)
              n1102 = Bundle By Name(cluster=w1566, "Integral Time (Ti, min)"=w1564) -> (w1565:T8)
              n1103 = local write "Stroke PID Gains"(w1565) -> ()
            }
            frame 17 {
              n1104 = local write "AIR TEMP INTERCEPT:"(w1567) -> ()
            }
            frame 18 {
              n1105 = local write "TEMP INTERCEPT:"(w1568) -> ()
            }
            frame 19 {
              n1106 = local write "S.NO"(w1569) -> ()
            }
            frame 20 {
              n1107 = local write "Com Port 3"(w1570) -> ()
            }
            frame 21 {
              n1108 = local write "LvdtOff"(w1571) -> ()
            }
            frame 22 {
              n1109 = local write "Humidity :"(w1572) -> ()
            }
            frame 23, Default {
            }
          }
        }
      }
    }
    n1110 = Select(t=u32 2500 ("milliseconds to wait"), s=w1519, f=u32 500 ("milliseconds to wait")) -> (s? t:f=w1517:u32)
    n1111 = Multiply(x=w1522, y=w1517) -> (x*y=w1524:dbl)
    n1112 = property on="FF Calibration g" class="WFGraph (strict)"("Visible"=w1513) -> ()  [unwired: 2 in, 2 out]
    n1113 = property on="Lift" class="Bool (strict)"("Visible"=w1513) -> ()  [unwired: 2 in, 2 out]
    n1114 = property on="Threshold" class="DigNum (strict)"("Visible"=w1513) -> ()  [unwired: 2 in, 2 out]
    n1115 = property on="Time slide" class="Slide (strict)"("Visible"=w1513) -> ()  [unwired: 2 in, 2 out]
    n1116 = call "Elapsed Time2"("Time Target (s)"=w1524, "Auto Reset"=TRUE) -> ("Time has Elapsed"=w1514:bool)  [unwired: 10 in, 7 out]
    n1117 = case shown="True" w1514 {
      frame False {
        # "79.77669138"
        # "2.3554"
        n1118 = local read "FRIC. FORCE :"() -> (w1577:dbl)
        n1119 = local read "FF cal val"() -> (w1574:dbl[])
        n1120 = Multiply(x=w1577, y=79.77669138) -> (x*y=w1576:dbl)
        n1121 = Multiply(x=w1574, y=w1576) -> (x*y=→"FF Calibration g":dbl[])
        "Err Count" <- 0 ("y")
      }
      frame True {
        n1122 = stacked-sequence {
          frame #0 {
            n1123 = stacked-sequence {
              frame #0 {
                "Lift" <- TRUE ("Lift")
              }
            }
          }
          frame #1 {
            w1589 = 2500 ("y")
            n1124 = local read "RUN"() -> (w1581:bool)
            n1125 = local read "FF1"() -> (w1584:dbl[])
            n1126 = case shown="False" w1581 {
              frame False {
                n1127 = local write "Frequency"(0.0 ("Frequency")) -> ()
              }
              frame True {
              }
            }
            n1128 = Array Size(array=w1584) -> (size(s)=w1583:i32)
            n1129 = local read "Ch1"() -> (w1580:dbl[])
            "Waveform Chart 2" <- w1580
            n1130 = call-poly <vilib>:"Mean.vi"("X"=w1580) -> ("mean"=→"Raw Mean":dbl)  [unwired: 1 out]
            n1131 = Insert Into Array(array=w1584, index=w1583, new element=w1580) -> (w1586:dbl[])
            n1132 = Array Size(array=w1586) -> (size(s)=w1590:i32)
            n1133 = Subtract(x=w1590, y=w1589) -> (x-y=w1588:i32)
            n1134 = Greater?(x=w1590, y=w1589) -> (0:w1591:bool)
            n1135 = case shown="True" w1591 {
              tunnel: w1588 -> [_ w1595]
              tunnel: [w1593 w1597] -> w1582
              tunnel: w1586 -> [w1593 w1596]
              frame False {
              }
              frame True {
                n1136 = Delete From Array(array=w1596, length=w1595, index=0) -> (array with subset deleted=w1597:dbl[])  [unwired: 1 out]
                "Numeric" <- w1595
              }
            }
            "FF1" <- w1582
            "PID Ref" <- TRUE ("PID Ref")
          }
          frame #2 {
          }
          frame #3 {
            w1605 = 0.0 ("lower limit")
            # "CONVERT TO N"
            # "DATA PROCESSING"
            # "115 mV/N"
            n1137 = local read "RH Numeric:"() -> (w1599:dbl)
            n1138 = local read "HUMIDITY:"() -> (w1600:dbl)
            n1139 = local read "temp buf"() -> (w1663:dbl[])
            n1140 = local read "Air temp"() -> (w1661:dbl[])
            n1141 = local read "ecr buf"() -> (w1622:dbl[])
            n1142 = local read "Fric Val"() -> (w1667:dbl[])
            n1143 = case shown="True" "Boolean 5" {
              frame False {
              }
              frame True {
                n1144 = local write "Boolean 5"(FALSE) -> ()
                n1145 = local write "Captured Values"(dbl[][] [] ("Captured Values")) -> ()
                n1146 = local write "Best Fit"(dbl[] [] ("Best Fit")) -> ()
              }
            }
            n1147 = local read "TEMPERATURE :"() -> (w1644:dbl)
            n1148 = call-poly <vilib>:"Mean.vi"("X"=w1622) -> ("mean"=w1619:dbl)  [unwired: 1 out]
            n1149 = call-poly <vilib>:"Mean.vi"("X"=w1661) -> ("mean"=w1629:dbl)  [unwired: 1 out]
            "Raw air temp" <- w1629
            n1150 = call-poly <vilib>:"Mean.vi"("X"=w1663) -> ("mean"=w1631:dbl)  [unwired: 1 out]
            "Raw specimen temp" <- w1631
            n1151 = local read "TEMP INTERCEPT:"() -> (w1636:dbl)
            n1152 = Multiply(x=w1599, y=w1600) -> (x*y=→"Humidity ( %RH )" →"Hum" →"Hum 2":dbl)
            n1153 = Multiply(x=w1667, y=1.0) -> (x*y=w1668:dbl[])
            n1154 = local read "FRIC. FORCE :"() -> (w1660:dbl)
            n1155 = Multiply(x=w1631, y=w1644) -> (x*y=w1625:dbl)
            n1156 = local read "AIR TEMPERATURE :"() -> (w1645:dbl)
            n1157 = local read "RUN"() -> (w1657:bool)
            n1158 = Add(x=w1629, y="Offset Air Temp") -> (x+y=w1624:dbl)
            n1159 = local read "AIR TEMP INTERCEPT:"() -> (w1641:dbl)
            n1160 = case shown="0, Default" "Calibrating" {
              tunnel: w1631 -> [w1687 _]
              tunnel: [w1687 w1688] -> w1630
              tunnel: w1629 -> [_ w1688]
              frame 0, Default {
              }
              frame 1 {
              }
            }
            n1161 = Multiply(x=w1619, y="ECR_Gain") -> (x*y=w1618:dbl)
            n1162 = Add(x=w1625, y=w1636) -> (x+y=w1642:dbl)
            n1163 = Multiply(x=w1660, y=79.77669138) -> (x*y=w1658:dbl)
            n1164 = Select(t=0.01 ("FF fil1"), s=w1657, f=0.1 ("FF fil1")) -> (s? t:f=w1653:dbl)
            n1165 = local read "ecr"() -> (w1613:dbl)
            n1166 = Multiply(x=w1624, y=w1645) -> (x*y=w1626:dbl)
            n1167 = Multiply(x=w1668, y=w1658) -> (x*y=w1665:dbl[])
            n1168 = Multiply(x=w1618, y=0.2) -> (x*y=w1611:dbl)
            n1169 = Multiply(x=0.8, y=w1613) -> (x*y=w1612:dbl)
            n1170 = call <vilib>:"Mean PtByPt.vi"("x"=w1642, "sample length"=10) -> ("mean"=w1601:dbl)  [unwired: 2 in, 1 out]
            "TEMP 2" <- w1601
            "TEMP 3" <- w1601
            n1171 = local read "AIR TEMP"() -> (w1650:dbl)
            n1172 = Add(x=w1626, y=w1641) -> (x+y=w1643:dbl)
            n1173 = call-poly <vilib>:"Mean.vi"("X"=w1665) -> ("mean"=w1666:dbl)  [unwired: 1 out]
            n1174 = Add(x=w1611, y=w1612) -> (x+y=w1610:dbl)
            n1175 = Subtract(x=1.0 ("y"), y=w1653) -> (x-y=w1651:dbl)
            n1176 = local write "TEMP"(w1601) -> ()
            n1177 = Multiply(x=w1651, y=w1650) -> (x*y=w1649:dbl)
            n1178 = Multiply(x=w1643, y=w1653) -> (x*y=w1654:dbl)
            n1179 = Not A Number/Path/Refnum?(number/path/refnum=w1610) -> (NaN/Path/Refnum?=w1620:bool)
            n1180 = Subtract(x=w1665, y=w1666) -> (x-y=w1635:dbl[])
            n1181 = local read "FRICVALZ"() -> (w1675:dbl)
            n1182 = case shown="True" "Boolean 4" {
              tunnel: w1630 -> [_ w1694]
              tunnel: "Standard Temp. ( °c )" -> [_ w1693]
              frame False {
              }
              frame True {
                n1183 = Build Array(w1693, w1694) -> (w1692:dbl[])
                n1184 = local write "Boolean 4"(FALSE ("Boolean 4")) -> ()
                n1185 = local read "Captured Values"() -> (w1691:dbl[][])
                n1186 = Build Array (concatenate)(w1691, w1692) -> (w1689:dbl[][])
                n1187 = local write "Captured Values"(w1689) -> ()
              }
            }
            n1188 = Or(x="FRICVALZ 3", y="FRICVALZ 2") -> (x .or. y?=w1603:bool)
            n1189 = Add(x=w1654, y=w1649) -> (x+y=w1647:dbl)
            n1190 = Absolute Value(x=w1635) -> (abs(x)=w1670:dbl[])
            n1191 = call-poly <vilib>:"RMS.vi"("X"=w1635) -> ("rms value"=w1634:dbl)  [unwired: 1 out]
            n1192 = Select(t=0.0, s=w1620, f=w1610) -> (s? t:f=w1617:dbl)
            n1193 = call-poly <vilib>:"Mean.vi"("X"=w1670) -> ()  [unwired: 2 out]
            n1194 = local read "FF 2"() -> (w1677:dbl)
            n1195 = case shown="True" w1603 {
              tunnel: w1634 -> [_ w1699]
              frame False {
              }
              frame True {
                w1698 = FALSE ("FRICVALZ")
                n1196 = local write "FRICVALZ 3"(w1698) -> ()
                n1197 = local write "FRICVALZ 2"(w1698) -> ()
                "FRICVALZ" <- w1699
              }
            }
            n1198 = Subtract(x=w1634, y=w1675) -> (x-y=w1669:dbl)
            n1199 = Not A Number/Path/Refnum?(number/path/refnum=w1647) -> (NaN/Path/Refnum?=w1648:bool)
            n1200 = In Range and Coerce(upper limit=100.0, x=w1617, lower limit=w1605) -> ()  [unwired: 2 out]
            n1201 = Select(t=0.0, s=w1648, f=w1647) -> (s? t:f=w1607:dbl)
            "AIR TEMP" <- w1607
            n1202 = Multiply(x=w1669, y=0.1 ("FF fil1")) -> (x*y=w1681:dbl)
            n1203 = Multiply(x=0.9 ("FF fil2"), y=w1677) -> (x*y=w1680:dbl)
            n1204 = call "Elapsed Time11"("Time Target (s)"=1.0) -> ("Time has Elapsed"=w1609:bool)  [unwired: 11 in, 7 out]
            n1205 = Add(x=w1681, y=w1680) -> (x+y=w1604:dbl)
            "FF 2" <- w1604
            "FF 4" <- w1604
            n1206 = local read "NORMAL LOAD"() -> (w1664:dbl)
            n1207 = case shown="True" w1609 {
              tunnel: w1607 -> [_ w1683]
              frame False {
              }
              frame True {
                "AirT" <- w1683
              }
            }
            n1208 = local read "TEMP"() -> (w1674:dbl)
            n1209 = Not A Number/Path/Refnum?(number/path/refnum=w1604) -> (NaN/Path/Refnum?=w1672:bool)
            n1210 = Divide(x=w1604, y=w1664) -> (x/y=w1637:dbl)
            n1211 = Not A Number/Path/Refnum?(number/path/refnum=w1674) -> (NaN/Path/Refnum?=w1673:bool)
            n1212 = Compound Arithmetic op=OR(w1673, w1672) -> (w1671:bool)
            n1213 = Not A Number/Path/Refnum?(number/path/refnum=w1637) -> (NaN/Path/Refnum?=w1639:bool)
            n1214 = case shown="True" w1671 {
              frame False {
              }
              frame True {
                n1215 = local write "TEMP"(0.0 ("TEMP")) -> ()
                n1216 = local write "FF 2"(0.0 ("FF 2")) -> ()
                n1217 = local write "reinit"(TRUE ("reinit")) -> ()
              }
            }
            n1218 = Select(t=0.0, s=w1639, f=w1637) -> (s? t:f=→"COF 2":dbl)
            "ecr" <- w1605
          }
          frame #4 {
            n1219 = case shown="True" "Boolean 6" {
              frame False {
              }
              frame True {
                n1220 = local write "Boolean 6"(FALSE ("Boolean 6")) -> ()
                n1221 = local read "Captured Values"() -> (w1710:dbl[][])
                n1222 = Index Array(array=w1710, index (col) #1=0 ("disabled index (col)"), index (col) #2=1 ("index (col)")) -> (element #1=w1708:dbl[], element #2=w1706:dbl[])  [unwired: 2 in]
                n1223 = call <vilib>:"Linear Fit.vi"("Y"=w1708, "X"=w1706) -> ("Best Linear Fit"=→"Best Fit":dbl[], "slope"=w1702:dbl, "intercept"=w1701:dbl)  [unwired: 9 in, 2 out]
                "Slope" <- w1702
                "Intercept" <- w1701
                n1224 = local read "Calibrating"() -> (w1703:u16)
                n1225 = case shown="1" w1703 {
                  tunnel: w1702 -> [w1712 w1714]
                  tunnel: w1701 -> [w1711 w1713]
                  frame 0, Default {
                    n1226 = local write "TEMPERATURE :"(w1712) -> ()
                    n1227 = local write "TEMP INTERCEPT:"(w1711) -> ()
                  }
                  frame 1 {
                    n1228 = local write "AIR TEMPERATURE :"(w1714) -> ()
                    n1229 = local write "AIR TEMP INTERCEPT:"(w1713) -> ()
                  }
                }
              }
            }
            n1230 = flat-sequence {
              frame #0 {
                n1231 = Wait (ms)(milliseconds to wait=u32 100) -> ()  [unwired: 1 out]
              }
              frame #1 {
                n1232 = local write "Lift"(FALSE ("Lift")) -> ()
              }
            }
          }
        }
      }
    }
    n1233 = Wait (ms)(milliseconds to wait=u32 50) -> ()  [unwired: 1 out]
    n1234 = local read "Quit"() -> (w1505:bool)
    "Rate" <- 2500.0 ("No of Samples")
    "Humid Last buf" <- dbl[] [0.0, 0.0, 0.0, 0.0] ("Humid Last buf")
  }
  n1235 = while {
    tunnel: w51 -> [_]
    tunnel: [w1744] -> _
    tunnel: [w1719] -> w48
    i -> [w1744]
    stop <- w1719 stop-if-true
    # "C:\\LAB-IQ-NXT\\Scar View.exe"
    n1236 = local read "OK Button 16"() -> (w1733:bool)
    n1237 = flat-sequence {
      frame #0 {
        n1238 = stacked-sequence {
          frame #0 {
            n1239 = local read "EDIT"() -> (w2398:bool)
            n1240 = case shown="True" w2398 {
              tunnel: [u8 2 ("Disabled") u8 0 ("Disabled")] -> _
              frame False {
                w2400 = FALSE
                n1241 = local write "Password"("") -> ()
                n1242 = property on="SrvM CP" class="Bool (strict)"("Visible"=w2400) -> ()  [unwired: 2 in, 2 out]
                n1243 = property on="message" class="Str"("Visible"=w2400) -> ()  [unwired: 2 in, 2 out]
                n1244 = local write "x = y?"(w2400) -> ()
                n1245 = property on="Password" class="Str"("Visible"=w2400) -> ()  [unwired: 2 in, 2 out]
                n1246 = property on="ENTER THE NEW PASSWORD" class="Str"("Visible"=w2400) -> ()  [unwired: 2 in, 2 out]
                n1247 = property on="ENTER CURRENT PASSWORD" class="Str"("Visible"=w2400) -> ()  [unwired: 2 in, 2 out]
                n1248 = local write "SrvM CP"(w2400) -> ()
              }
              frame True {
                w2403 = TRUE
                n1249 = property on="SrvM CP" class="Bool (strict)"("Visible"=w2403) -> ()  [unwired: 2 in, 2 out]
                n1250 = property on="Password" class="Str"("Visible"=w2403) -> ()  [unwired: 2 in, 2 out]
              }
            }
            "dipl pwd" <- "@143$\n" ("dipl pwd")
          }
          frame #1 {
            # "Gain password"
            n1251 = String To Byte Array(string="ENTER CURRENT PASSWORD") -> (unsigned byte array=w2408:u8[])
            n1252 = Search 1D Array(1D array=w2408, element=u8 10) -> (index of element=w2411:i32)  [unwired: 1 in]
            n1253 = Index Array(array=w2408, index=w2411) -> (element=w2407:u8)
            n1254 = Equal?(x=w2407, y=10) -> (x = y?=w2405:bool)
            n1255 = case shown="True" w2405 {
              frame False {
